vi "celsius to farenheit.vi"(0 "Temperature in Degree Celsius":dbl) -> (4 "Temperature in Farenheit":dbl)   [LabVIEW 2018]
panel:
  # "This application will convert temperature values in Degrees to Farenheit"
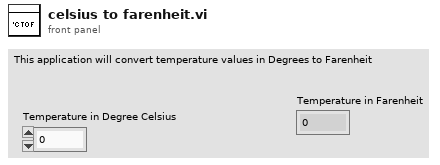
[diagram p1: front panel]
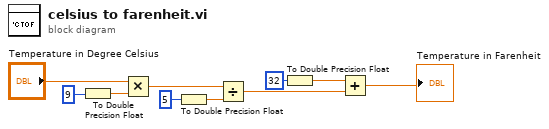
[diagram p0: block diagram]
diagram:
  n1 = To Double Precision Float(number=9) -> (double precision float=w6:dbl)
  n2 = Multiply(x="Temperature in Degree Celsius", y=w6) -> (x*y=w9:dbl)
  n3 = To Double Precision Float(number=5) -> (double precision float=w4:dbl)
  n4 = Divide(x=w9, y=w4) -> (x/y=w8:dbl)
  n5 = To Double Precision Float(number=32) -> (double precision float=w2:dbl)
  n6 = Add(x=w2, y=w8) -> (x+y=→"Temperature in Farenheit":dbl)
